vi "Write Topics.vi"(8 "error in":errorcluster, 10 "Topics":T1[](array[typedef]), 11 "System in":refnum<class "System.lvclass">) -> (0 "error out":errorcluster, 3 "System out":refnum<class "System.lvclass">)   [LabVIEW 2014, in "System.lvclass"]
uses:
  System.lvclass
  Controls/Topic Ref.ctl
  System.lvclass/System.ctl
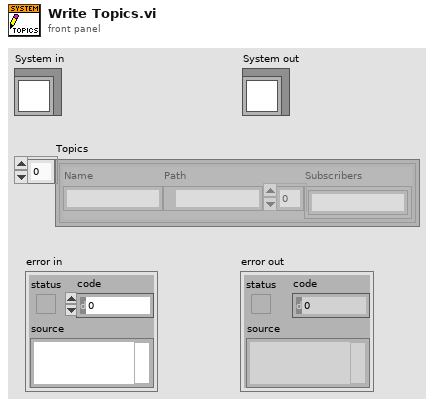
[diagram p1: front panel]
types:
  T1 = typedef "Topic Ref.ctl" = cluster{"Name":string, "Path":path, "Subscribers":string[]}
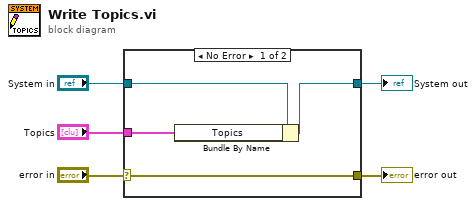
[diagram p0: block diagram]
diagram:
  n1 = case shown="No Error" "error in" {
    selector: "error in" -> [w9 w10]
    tunnel: [w9 w10] -> w4
    tunnel: [w7 w11] -> w2
    tunnel: "System in" -> [w8 w11]
    tunnel: "Topics" -> [w6 _]
    frame No Error {
      n2 = Bundle By Name(cluster=w8, "Topics"=w6) -> (w7:refnum<class "System.lvclass">)
    }
    frame Error {
    }
  }
  "error out" <- w4
  "System out" <- w2
